vi "Redraw Tree.vi"(8 "error in (no error)":errorcluster, 11 "Actor Monitor in":refnum<class "Actor Monitor.lvclass">) -> (0 "error out":errorcluster, 3 "Actor Monitor out":refnum<class "Actor Monitor.lvclass">)   [LabVIEW 2018, in "Monitored Actor.lvlib" / "Actor Monitor.lvclass"]
doc: "Parses the memory structors and builds a tree representation of the launched actor\n\nCopyright: MGI\nAuthored by: Derek Trepanier"
uses:
  Actor Monitor.lvclass
  <vilib>/ActorFramework/Message Enqueuer/Message Enqueuer.lvclass
  UI Info.ctl
  Actor Monitor.lvclass/Actor Monitor.ctl
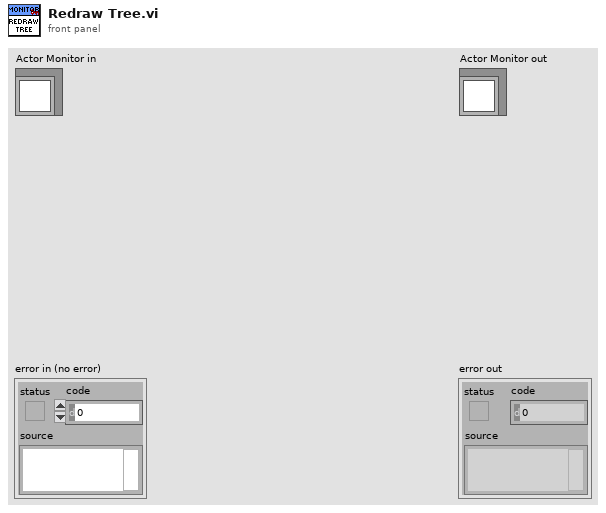
[diagram p1: front panel]
types:
  T1 = typedef "Monitored Actor.lvlib/Actor Monitor.lvclass/UI Info.ctl" = cluster{"Class Name":string, "Actor Core Name":string, "Ping Response Str":string}
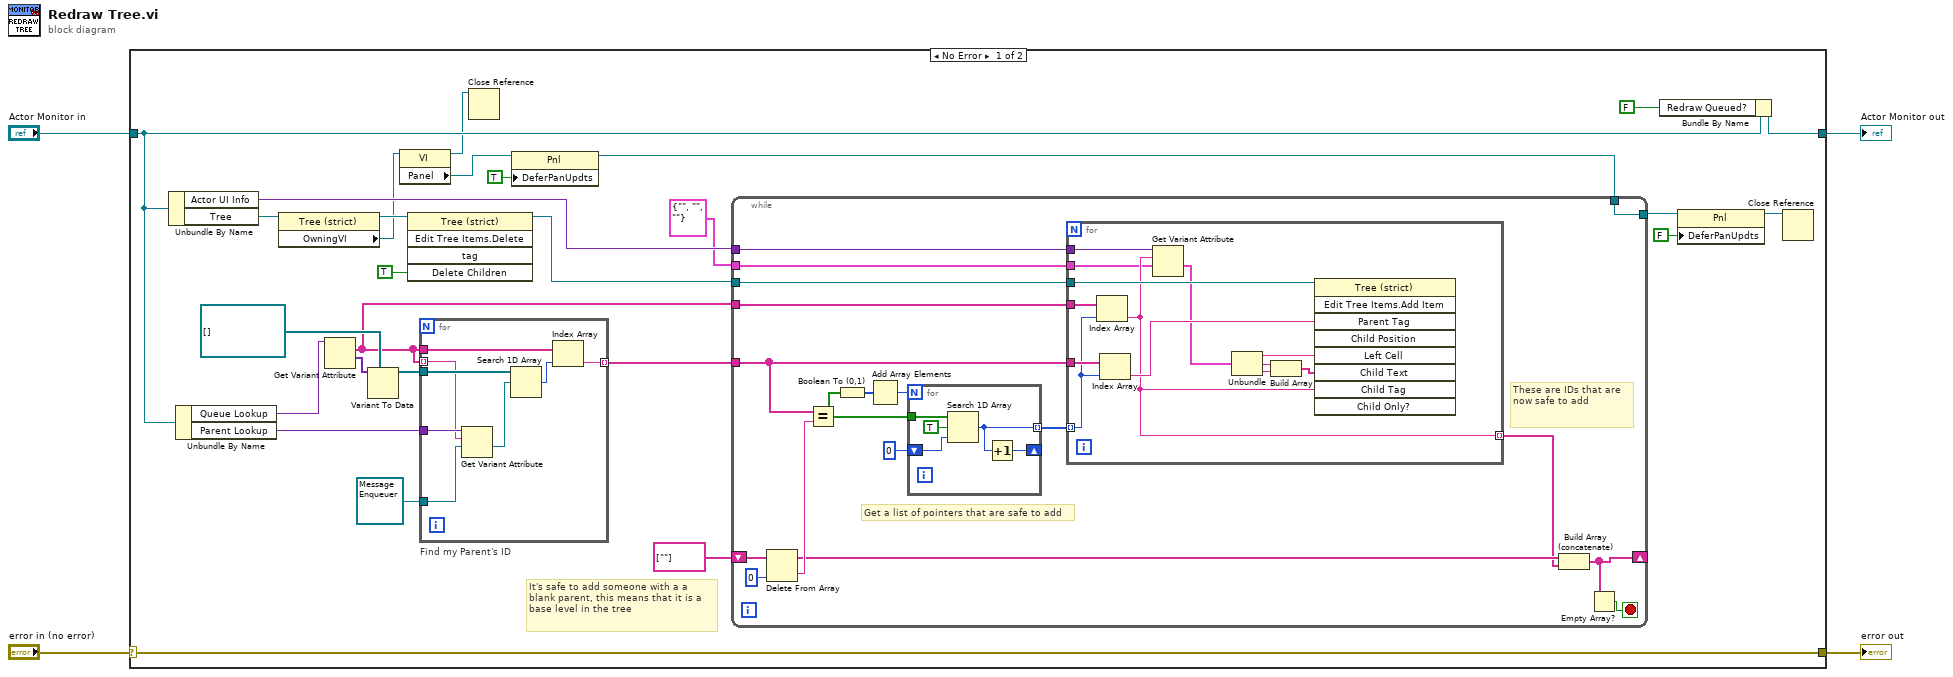
[diagram p0: block diagram]
diagram:
  n1 = case shown="No Error" "error in (no error)" {
    selector: "error in (no error)" -> [w31 w77]
    tunnel: [w31 w77] -> w3
    tunnel: [w15 w76] -> w1
    tunnel: "Actor Monitor in" -> [w24 w76]
    frame No Error {
      # "It's safe to add someone with a a blank parent, this means that it is a base level in the tree"
      n2 = Unbundle By Name(w24) -> ("Actor UI Info"=w20:variant, "Tree"=w21:refnum<vi>)
      n3 = Unbundle By Name(w24) -> ("Queue Lookup"=w30:variant, "Parent Lookup"=w27:variant)
      n4 = property class="Tree (strict)"(reference=w21) -> (reference out=w13:refnum<vi>, "OwningVI"=w12:refnum<vi>)  [unwired: 1 in, 1 out]
      n5 = Get Variant Attribute(Variant=w30) -> (names=w23:string[], values=w29:variant[])  [unwired: 3 in, 2 out]
      n6 = Variant To Data(type=refnum<class "Message Enqueuer.lvclass">[] [], Variant=w29) -> (data=w25:refnum<class "Message Enqueuer.lvclass">[])  [unwired: 1 in, 1 out]
      n7 = property class="VI"(reference=w12) -> (reference out=w10:refnum<vi>, "Panel"=w11:refnum<vi>)  [unwired: 1 in, 1 out]
      n8 = invoke class="Tree (strict)" method="Edit Tree Items.Delete"(reference=w13, "Delete Children"=TRUE ("Delete Children?")) -> (reference out=w19:refnum<vi>)  [unwired: 3 in, 4 out]
      n9 = for "Find my Parent's ID" {
        tunnel: w23 -> [w70]
        tunnel: w27 -> [w75]
        tunnel: refnum<class "Message Enqueuer.lvclass"> refnum ("Caller Enqueuer") -> [w74]
        tunnel: w25 -> [w73]
        tunnel: w23 -> [w71] mode=indexing
        tunnel: [w68] -> w22 mode=indexing
        n10 = Get Variant Attribute(Variant=w75, name=w71, default value (empty Variant)=w74) -> (value=w72:refnum<class "Message Enqueuer.lvclass">)  [unwired: 1 in, 3 out]
        n11 = Search 1D Array(1D array=w73, element=w72) -> (index of element=w69:i32)  [unwired: 1 in]
        n12 = Index Array(array=w70, index=w69) -> (element=w68:string)
      }
      n13 = Close Reference(reference=w10) -> ()  [unwired: 1 in, 1 out]
      n14 = property class="Pnl"(reference=w11, "DeferPanUpdts"=TRUE ("Defer Panel Updates")) -> (reference out=w8:refnum<vi>)  [unwired: 1 in, 1 out]
      n15 = while {
        tunnel: w23 -> [w45]
        tunnel: w22 -> [w43]
        tunnel: w20 -> [w42]
        tunnel: w19 -> [w41]
        shift-right: [w34] -> _
        shift-left: string[] [""] -> [w40]
        tunnel: T1 {"Class Name"="", "Actor Core Name"="", "Ping Response Str"=""} ("UI Info") -> [w33]
        tunnel: [w32] -> w7
        tunnel: w8 -> [w32]
        stop <- w35 stop-if-true
        # "These are IDs that are now safe to add"
        # "Get a list of pointers that are safe to add"
        n16 = Delete From Array(array=w40, index=0) -> (deleted portion=w39:string, array with subset deleted=w38:string[])  [unwired: 1 in]
        n17 = Equal?(x=w43, y=w39) -> (x = y?=w47:bool[])
        n18 = Boolean To (0,1)(Boolean=w47) -> (0, 1=w48:i16[])
        n19 = Add Array Elements(numeric array=w48) -> (sum=w49:i16)
        n20 = for {
          N: w49 -> [_]
          tunnel: w47 -> [w67]
          tunnel: [w65] -> w44 mode=indexing
          shift-right: [w63] -> _
          shift-left: 0 ("index of element") -> [w64]
          n21 = Search 1D Array(1D array=w67, element=TRUE, start index (0)=w64) -> (index of element=w65:i32)
          n22 = Increment(x=w65) -> (x+1=w63:i32)
        }
        n23 = for {
          tunnel: w45 -> [w59]
          tunnel: w44 -> [w57] mode=indexing
          tunnel: w43 -> [w61]
          tunnel: w41 -> [w62]
          tunnel: w42 -> [w58]
          tunnel: [w56] -> w37 mode=indexing
          tunnel: w33 -> [w55]
          n24 = Index Array(array=w59, index=w57) -> (element=w56:string)
          n25 = Index Array(array=w61, index=w57) -> (element=w60:string)
          n26 = Get Variant Attribute(Variant=w58, name=w56, default value (empty Variant)=w55) -> (value=w54:T1)  [unwired: 1 in, 3 out]
          n27 = Unbundle(w54) -> ("Class Name"=w53:string, "Actor Core Name"=w52:string, "Ping Response Str"=w51:string)
          n28 = Build Array(w52, w51) -> (w50:string[])
          n29 = invoke class="Tree (strict)" method="Edit Tree Items.Add Item"(reference=w62, "Parent Tag"=w60, "Left Cell"=w53, "Child Text"=w50, "Child Tag"=w56) -> ()  [unwired: 4 in, 9 out]
        }
        n30 = Build Array (concatenate)(w38, w37) -> (w34:string[])
        n31 = Empty Array?(array=w34) -> (empty?=w35:bool)
      }
      n32 = Bundle By Name(cluster=w24, "Redraw Queued?"=FALSE ("Tree out of date?")) -> (w15:refnum<class "Actor Monitor.lvclass">)
      n33 = property class="Pnl"(reference=w7, "DeferPanUpdts"=FALSE ("Defer Panel Updates")) -> (reference out=w5:refnum<vi>)  [unwired: 1 in, 1 out]
      n34 = Close Reference(reference=w5) -> ()  [unwired: 1 in, 1 out]
    }
    frame Error {
    }
  }
  "error out" <- w3
  "Actor Monitor out" <- w1
